vi "To JSON.vi"(5 "enable LabVIEW extensions? (T)":bool=TRUE, 6 "Pretty Print?":bool, 7 "LVClass Serializer":refnum<class "JSONtext LVClass Serializer.lvclass">, 8 "error in (no error)":errorcluster, 11 "Recursive JSON Serializable in":refnum<class "Recursive JSON Serializable.lvclass">) -> (0 "error out":errorcluster, 2 "<JSON>":string, 3 "Recursive JSON Serializable out":refnum<class "Recursive JSON Serializable.lvclass">)   [LabVIEW 2017, in "JSON Serializable Serializer Tests.lvlib" / "Recursive JSON Serializable.lvclass"]
doc: "Creates a JSON string from an object."
uses:
  Recursive JSON Serializable.lvclass
  <vilib>/JDP Science/JSONtext/LVClass Serializer/JSONtext LVClass Serializer.lvclass
  Recursive JSON Serializable.lvclass/Recursive JSON Serializable.ctl
  <vilib>/JDP Science/JSONtext/JSONtext.lvlib
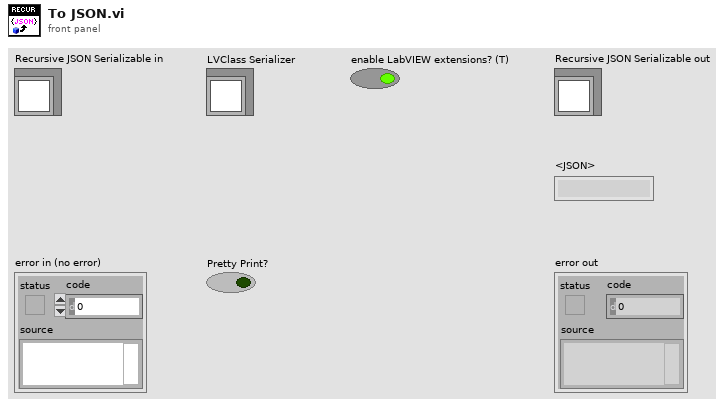
[diagram p1: front panel]
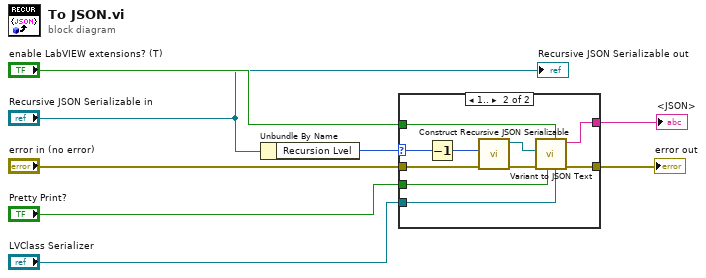
[diagram p0: block diagram]
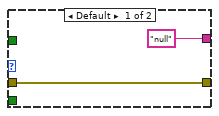
[diagram p2: hidden frame]
diagram:
  n1 = Unbundle By Name("Recursive JSON Serializable in") -> ("Recursion Lvel"=w1:u8)
  n2 = case shown="1.." w1 {
    selector: w1 -> [_ w12]
    tunnel: [w9 w20] -> w8
    tunnel: "enable LabVIEW extensions? (T)" -> [_ w19]
    tunnel: "Pretty Print?" -> [_ w18]
    tunnel: "LVClass Serializer" -> [_ w17]
    tunnel: ["null" ("<JSON>") w16] -> w4
    tunnel: "error in (no error)" -> [w9 w15]
    frame Default {
    }
    frame 1.. {
      n3 = Decrement(x=w12) -> (x-1=w13:u8)
      n4 = call "Construct Recursive JSON Serializable.vi"("error in (no error)"=w15, "Recursion Level"=w13) -> ("error out"=w14:errorcluster, "Recursive JSON Serializable"=w11:refnum<class "Recursive JSON Serializable.lvclass">)  [unwired: 8 in]
      n5 = call <vilib>:"Variant to JSON Text.vi"("LVClass Serializer"=w17, "enable LabVIEW extensions? (T)"=w19, "Pretty Print?"=w18, "error in (no error)"=w14, "Variant"=w11) -> ("error out"=w20:errorcluster, "<JSON>"=w16:string)  [unwired: 4 in, 1 out]
    }
  }
  "error out" <- w8
  "<JSON>" <- w4
  "Recursive JSON Serializable out" <- "Recursive JSON Serializable in"
